vi "func1 (SubVI).vi"(1 "input in":i32) -> (0 "input out":i32)   [LabVIEW 2014]
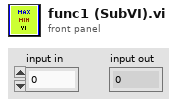
[diagram p1: front panel]
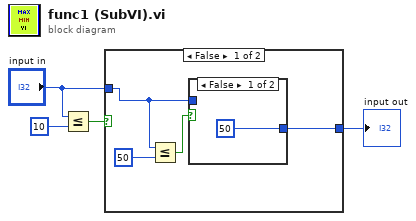
[diagram p0: block diagram]
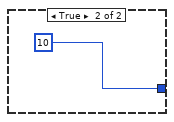
[diagram p3: hidden frame]
diagram:
  n1 = Less Or Equal?(x="input in", y=10) -> (x <= y?=w2:bool)
  n2 = case shown="False" w2 {
    tunnel: [w6 10] -> w4
    tunnel: "input in" -> [w5 _]
    frame False {
      n3 = Less Or Equal?(x=w5, y=50) -> (x <= y?=w7:bool)
      n4 = case shown="False" w7 {
        tunnel: [50 w10] -> w6
        tunnel: w5 -> [_ w10]
        frame False {
        }
        frame True {
        }
      }
    }
    frame True {
    }
  }
  "input out" <- w4
